vi "Parse-Build_Tile_Array.vi"(9 "Rows":T3[](array[typedef]), 10 "Barrier Coords":T2[](array[typedef]), 11 "Columns":T3[](array[typedef])) -> (2 "output array":T1[][](array[typedef]))   [LabVIEW 2020]
uses:
  Controls/Scan_Values.ctl
  Controls/Parse-(X,Y).ctl
  Controls/TileColor.ctl
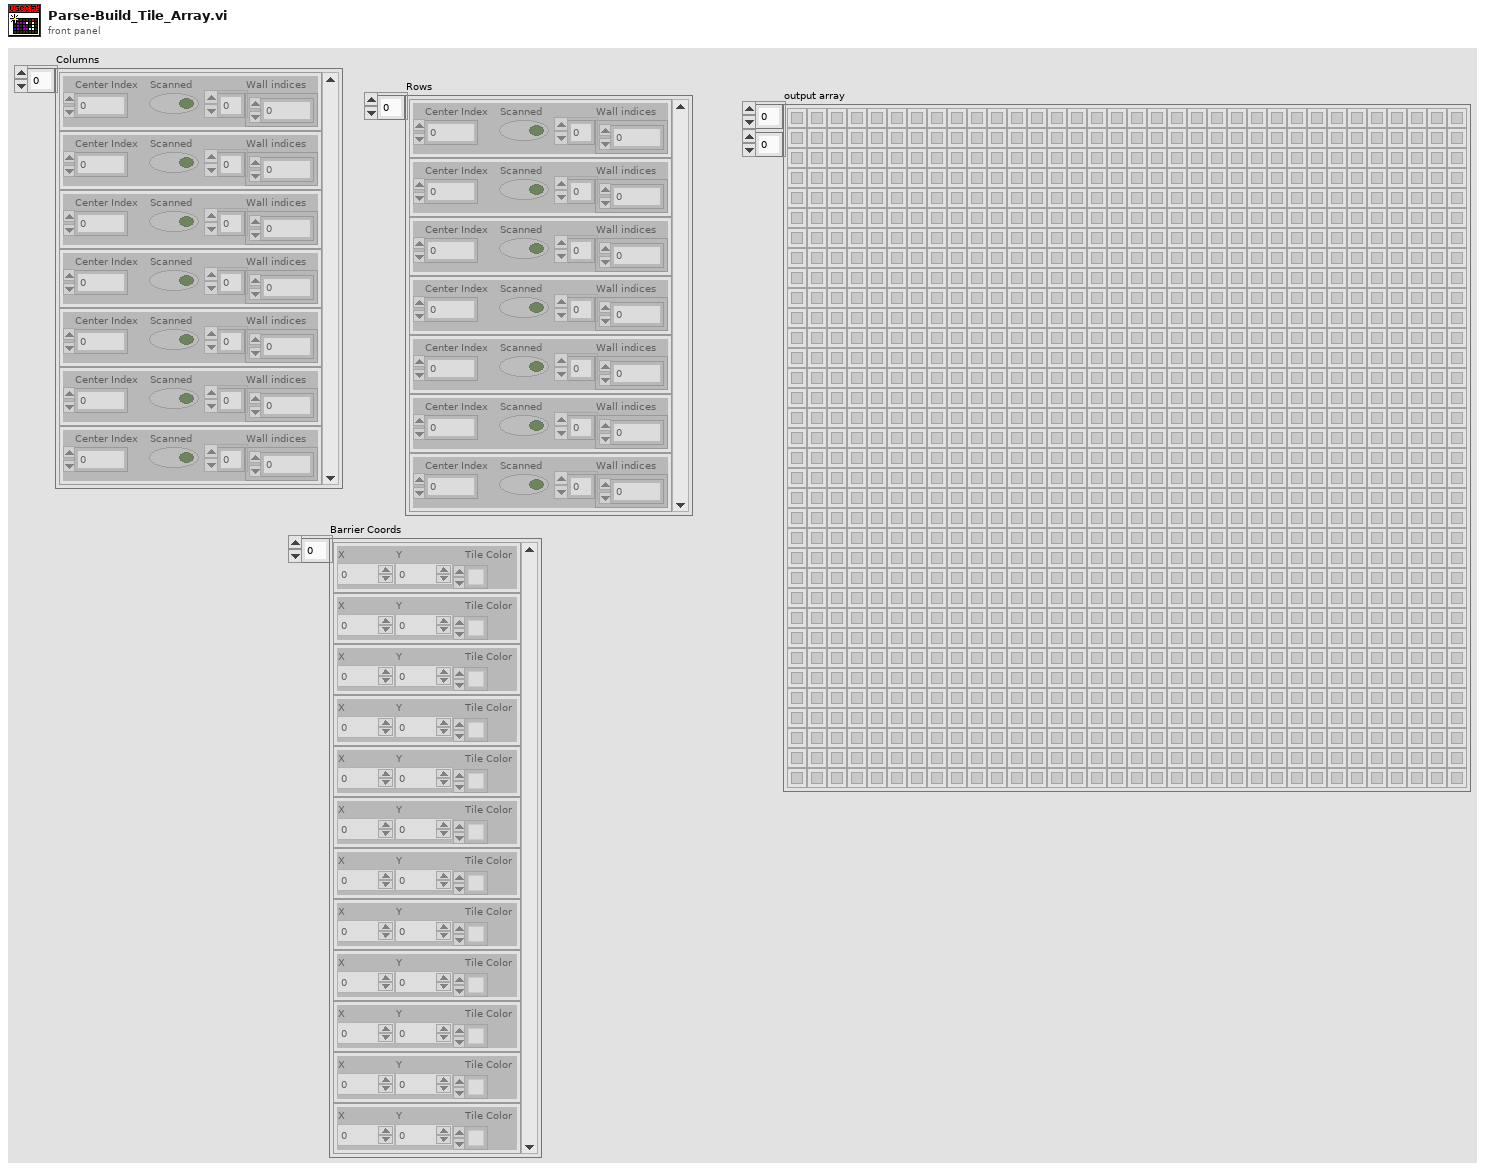
[diagram p1: front panel]
types:
  T1 = typedef "TileColor.ctl" = u16
  T2 = typedef "Parse-(X,Y).ctl" = cluster{"X":i32, "Y":i32, "Tile Color":T1}
  T3 = typedef "Scan_Values.ctl" = cluster{"Center Index":i32, "Scanned":bool, "Wall indices":i32[]}
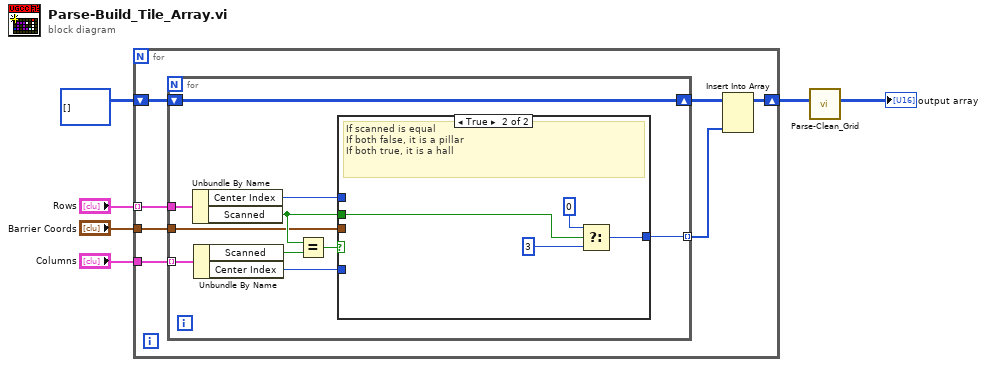
[diagram p0: block diagram]
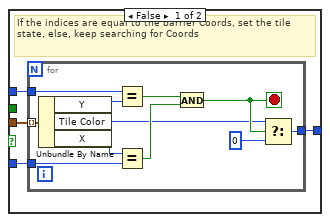
[diagram p2: hidden frame]
diagram:
  n1 = for {
    tunnel: "Rows" -> [w13] mode=indexing
    tunnel: "Columns" -> [w12]
    tunnel: "Barrier Coords" -> [w11]
    shift-right: [w7] -> w2
    shift-left: T1[][] [] -> [w10]
    n2 = for {
      tunnel: w13 -> [w23]
      tunnel: w12 -> [w22] mode=indexing
      tunnel: [w21] -> w8 mode=indexing
      tunnel: w11 -> [w18]
      shift-right: [w15] -> w9
      shift-left: w10 -> [w15]
      n3 = Unbundle By Name(w23) -> ("Center Index"=w16:i32, "Scanned"=w19:bool)
      n4 = Unbundle By Name(w22) -> ("Scanned"=w14:bool, "Center Index"=w17:i32)
      n5 = Equal?(x=w19, y=w14) -> (x = y?=w20:bool)
      n6 = case shown="True" w20 {
        tunnel: [w24 w42] -> w21
        tunnel: w19 -> [_ w39]
        tunnel: w18 -> [w27 _]
        tunnel: w17 -> [w26 _]
        tunnel: w16 -> [w25 _]
        frame False {
          # "If the indices are equal to the barrier Coords, set the tile\nstate, else, keep searching for Coords"
          n7 = for {
            tunnel: w27 -> [w38] mode=indexing
            tunnel: w26 -> [w37]
            tunnel: w25 -> [w35]
            tunnel: [w31] -> w24
            stop <- w32 stop-if-true
            n8 = Unbundle By Name(w38) -> ("Y"=w36:i32, "Tile Color"=w29:T1, "X"=w28:i32)
            n9 = Equal?(x=w35, y=w36) -> (x = y?=w34:bool)
            n10 = Equal?(x=w28, y=w37) -> (x = y?=w33:bool)
            n11 = And(x=w34, y=w33) -> (x .and. y?=w32:bool)
            n12 = Select(t=w29, s=w32, f=T1 0 ("Tile")) -> (s? t:f=w31:T1)
          }
        }
        frame True {
          # "If scanned is equal\nIf both false, it is a pillar\nIf both true, it is a hall"
          n13 = Select(t=T1 0 ("Tile"), s=w39, f=T1 3 ("Tile")) -> (s? t:f=w42:T1)
        }
      }
    }
    n14 = Insert Into Array(array=w9, new element=w8) -> (w7:T1[][])  [unwired: 2 in]
  }
  n15 = call "Parse-Clean_Grid.vi"("Tile Array"=w2) -> ("Cleaned Maze"=→"output array":T1[][])  [unwired: 10 in]
